vi "Remove.vi"(8 "error in (no error)":errorcluster, 10 "Index":i32, 11 "ListImp in":refnum<class "ListImp.lvclass">) -> (0 "error out":errorcluster, 1 "Item":refnum<class>, 3 "ListImp out":refnum<class "ListImp.lvclass">)   [LabVIEW 2013, in "LapDog.Collections.v_.Lists.lvlib" / "ListImp.lvclass"]
doc: "Removes an item from the list at the given Index. An Index of -1 removes the last item in the list. If no item exists at the given Index error 510201 is returned."
uses:
  ListImp.lvclass
  LapDog.Collections.Common/LapDog.Collections.v_.Common.lvlib
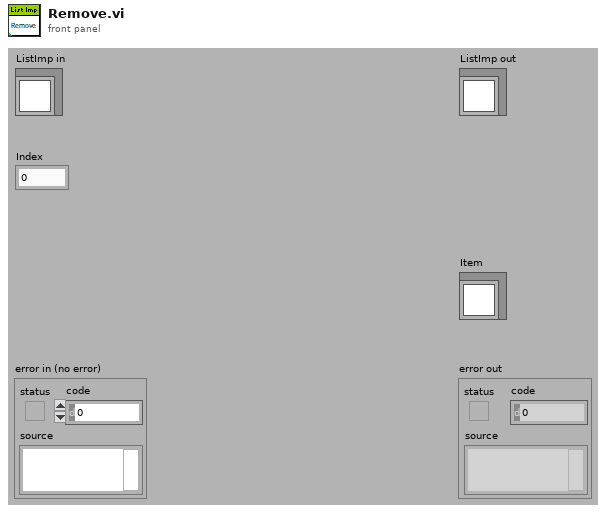
[diagram p1: front panel]
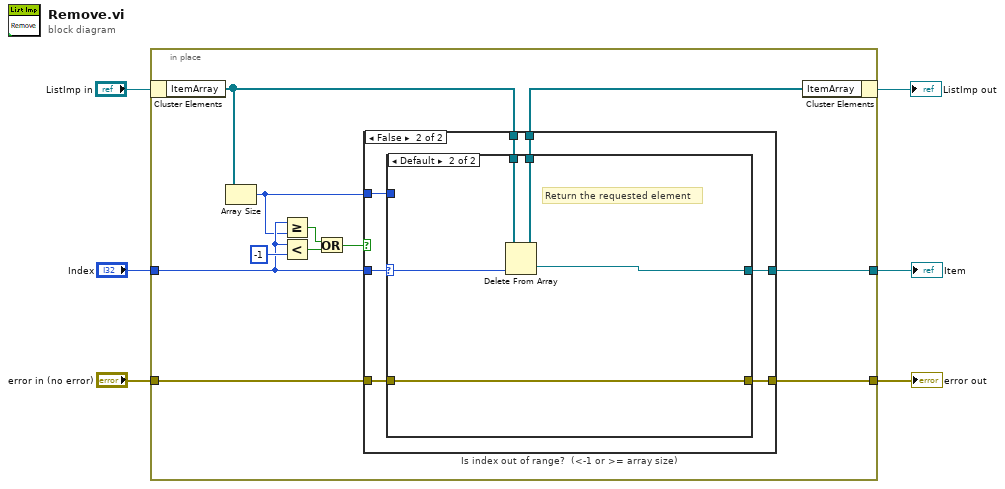
[diagram p0: block diagram]
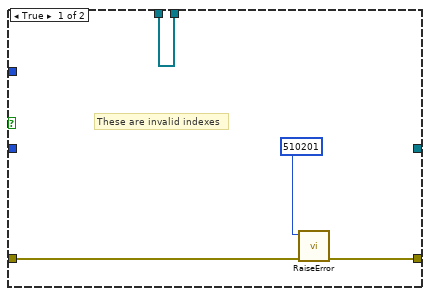
[diagram p2: hidden frame]
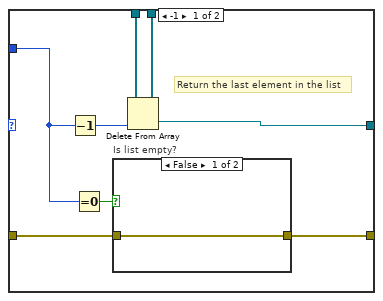
[diagram p3: hidden frame]
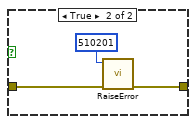
[diagram p4: hidden frame]
diagram:
  n1 = in-place {
    in-place-border: [w17] -> w1
    in-place-border: "error in (no error)" -> [w16]
    in-place-border: [w15] -> w2
    in-place-border: "Index" -> [w10]
    n2 = in-place-cluster #1("ListImp in") -> ("ItemArray"=w9:refnum<class>[])
    n3 = Array Size(array=w9) -> (size(s)=w7:i32)
    n4 = Greater Or Equal?(x=w10, y=w7) -> (x >= y?=w12:bool)
    n5 = Less?(x=w10, y=-1) -> (x < y?=w13:bool)
    n6 = Or(x=w12, y=w13) -> (x .or. y?=w11:bool)
    n7 = case "Is index out of range?  (<-1 or >= array size)" shown="False" w11 {
      tunnel: [_ w28] -> w17
      tunnel: w9 -> [w18 w27]
      tunnel: w16 -> [w21 w22]
      tunnel: [w20 w23] -> w15
      tunnel: w10 -> [_ w26]
      tunnel: [w18 w25] -> w8
      tunnel: w7 -> [_ w24]
      frame True {
        # "These are invalid indexes"
        n8 = call "RaiseError.vi"("error in (no error)"=w21, "Error Code"=510201) -> ("error out"=w20:errorcluster)  [unwired: 9 in]
      }
      frame False {
        n9 = case shown="Default" w26 {
          selector: w26 -> [_ w43]
          tunnel: [w36 w45] -> w28
          tunnel: w27 -> [w35 w44]
          tunnel: [w33 w42] -> w25
          tunnel: w24 -> [w29 _]
          tunnel: [w31 w41] -> w23
          tunnel: w22 -> [w32 w41]
          frame -1 {
            # "Return the last element in the list"
            n10 = Decrement(x=w29) -> (x-1=w34:i32)
            n11 = Equal To 0?(x=w29) -> (x = 0?=w30:bool)
            n12 = case "Is list empty?" shown="False" w30 {
              tunnel: w32 -> [w37 w39]
              tunnel: [w37 w38] -> w31
              frame False {
              }
              frame True {
                n13 = call "RaiseError.vi"("error in (no error)"=w39, "Error Code"=510201) -> ("error out"=w38:errorcluster)  [unwired: 9 in]
              }
            }
            n14 = Delete From Array(array=w35, index=w34) -> (deleted portion=w36:refnum<class>, array with subset deleted=w33:refnum<class>[])  [unwired: 1 in]
          }
          frame Default {
            # "Return the requested element"
            n15 = Delete From Array(array=w44, index=w43) -> (deleted portion=w45:refnum<class>, array with subset deleted=w42:refnum<class>[])  [unwired: 1 in]
          }
        }
      }
    }
    n16 = in-place-cluster #1("ItemArray"=w8) -> (→"ListImp out":refnum<class "ListImp.lvclass">)
  }
  "error out" <- w2
  "Item" <- w1
